vi "Add.vi"(8 "error in":errorcluster, 9 "Value":refnum<class "Value.lvclass">, 10 "Key":refnum<class "Key Name.lvclass">, 11 "Supported Objects in":refnum<class "Supported Objects.lvclass">) -> (0 "error out":errorcluster, 3 "Supported Objects out":refnum<class "Supported Objects.lvclass">)   [LabVIEW 2019, in "Electronic Datasheet.lvlib" / "Supported Objects.lvclass"]
uses:
  Supported Objects.lvclass
  Supported Objects.lvclass/Supported Objects.ctl
  Keyname/Key Name.lvclass
  Electronic Datasheet.lvlib
  Value/Value.lvclass
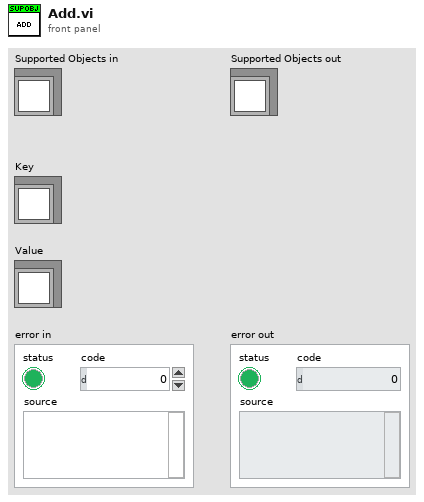
[diagram p1: front panel]
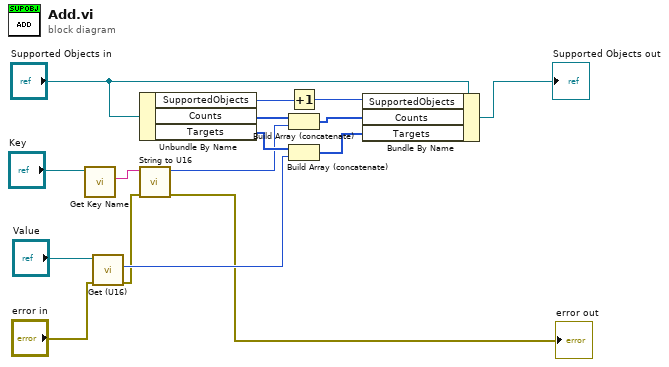
[diagram p0: block diagram]
diagram:
  n1 = call "Get Key Name.vi"("Key Name in"="Key") -> ("Keyname"=w5:string)  [unwired: 9 in, 1 out]
  n2 = call "Get (U16).vi"("error in"="error in", "Value in"="Value") -> ("error out"=w1:errorcluster, "Value"=w8:u16)  [unwired: 6 in, 2 out]
  n3 = Unbundle By Name("Supported Objects in") -> ("SupportedObjects"=w4:u16, "Counts"=w14:u16[], "Targets"=w12:u16[])
  n4 = call "String to U16.vi"("error in"=w1, "Integer String"=w5) -> ("error out"=→"error out":errorcluster, "U16"=w10:u16)  [unwired: 8 in]
  n5 = Increment(x=w4) -> (x+1=w3:u16)
  n6 = Build Array (concatenate)(w14, w10) -> (w13:u16[])
  n7 = Build Array (concatenate)(w12, w8) -> (w11:u16[])
  n8 = Bundle By Name(cluster="Supported Objects in", "SupportedObjects"=w3, "Counts"=w13, "Targets"=w11) -> (→"Supported Objects out":refnum<class "Supported Objects.lvclass">)
